vi "RW.vi"(2 "button":string, 3 "address string":string) -> (0 "out":string, 1 "number":dbl format="%#.6p")   [LabVIEW 2017]
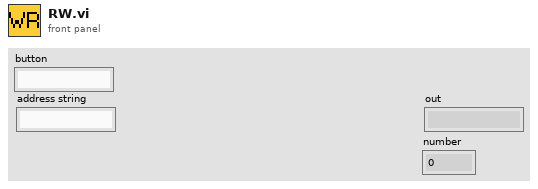
[diagram p1: front panel]
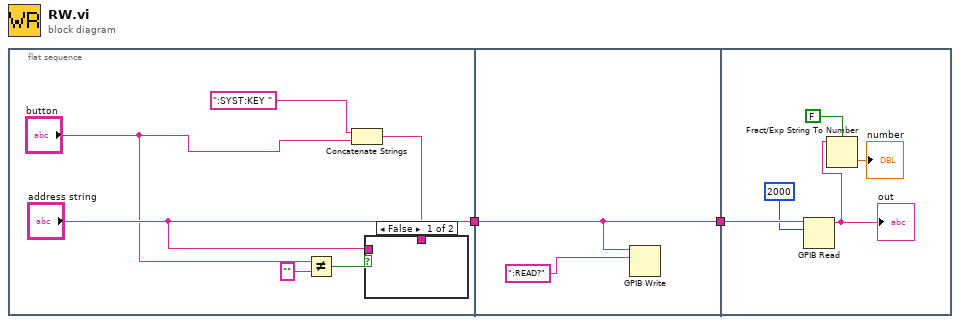
[diagram p0: block diagram]
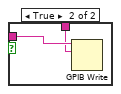
[diagram p2: hidden frame]
diagram:
  n1 = flat-sequence {
    tunnel: ["address string"] -> w2
    tunnel: w2 -> [w12]
    tunnel: [w12] -> w1
    tunnel: w1 -> [w17]
    frame #0 {
      n2 = Not Equal?(x="button", y="") -> (x != y?=w5:bool)
      n3 = Concatenate Strings(":SYST:KEY " ("string"), "button") -> (w7:string)
      n4 = case shown="False" w5 {
        tunnel: "address string" -> [_ w10]
        tunnel: w7 -> [_ w9]
        frame False {
        }
        frame True {
          n5 = GPIB Write(0:w10, 1:w9) -> ()  [unwired: 3 in, 2 out]
        }
      }
    }
    frame #1 {
      n6 = GPIB Write(0:w12, 1:":READ?" ("string")) -> ()  [unwired: 3 in, 2 out]
    }
    frame #2 {
      n7 = GPIB Read(0:w17, 1:2000 ("timeout ms (488.2 global)")) -> (5:w15:string)  [unwired: 3 in, 2 out]
      "out" <- w15
      n8 = Fract/Exp String To Number(use system decimal point (T)=FALSE, string=w15) -> (number=→"number":dbl)  [unwired: 2 in, 1 out]
    }
  }
